vi "PM-A-Serial-test_setup.vi"() -> ()   [LabVIEW 2018]
uses:
  <vilib>/measure/matone.llb/Extract Single Tone Information 1 Chan.vi
  <vilib>/measure/NI_MAPro.lvlib
panel:
  out "Pulse":dbl format="%.2p"
  out "x-y":u32
  in  "sample rate [Hz] (1000)":dbl=1000.0
  out "error out":errorcluster
  out "Filter":waveform(dbl)(graph)
  in  "Addition signal to remove (0) [s]":dbl
  in  "Clear data":bool
  in  "Samples s":i32=10
  out "Raw":waveform(dbl)(graph)
  in  "Stop":bool
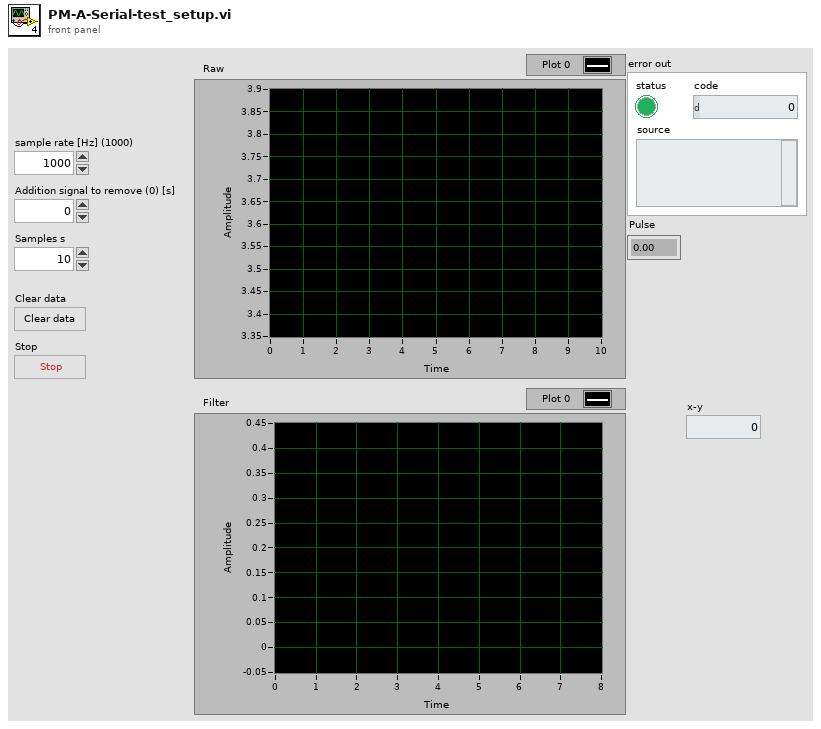
[diagram p1: front panel]
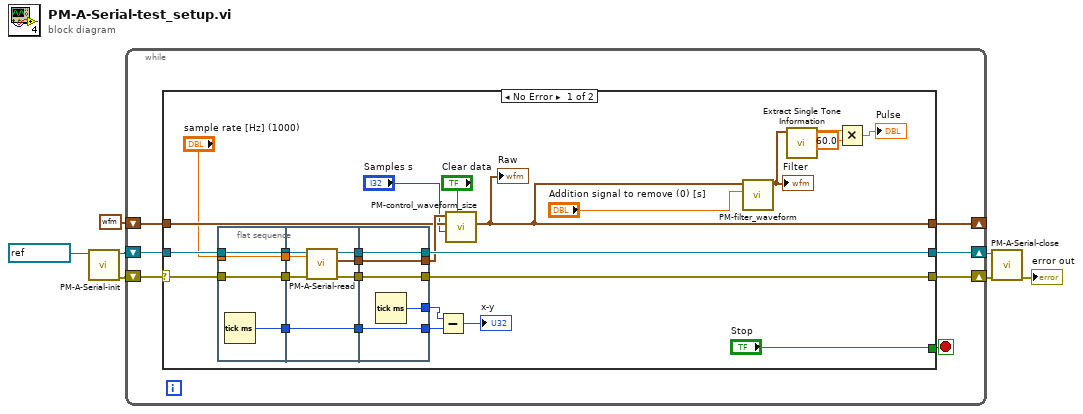
[diagram p0: block diagram]
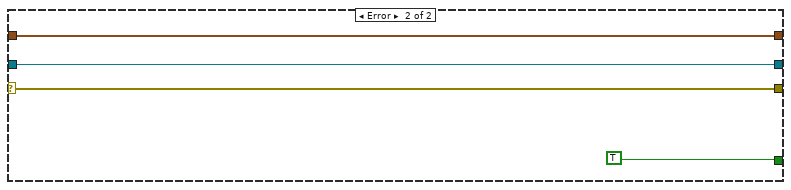
[diagram p2: hidden frame]
diagram:
  n1 = call "PM-A-Serial-init.vi"("VISA resource name"=refnum<visa-resource-name> "COM5" ("VISA resource name in")) -> ("error out"=w7:errorcluster, "VISA resource name out"=w6:refnum<visa-resource-name>)  [unwired: 9 in]
  n2 = while {
    shift-right: [w14] -> w2
    shift-left: w7 -> [w13]
    shift-right: [w12] -> w3
    shift-left: w6 -> [w11]
    shift-right: [w9] -> _
    shift-left: waveform(dbl) {"t0"=timestamp(0 s since 1904-01-01), "dt"=1.0, "Y"=[]} ("data") -> [w10]
    stop <- w8 stop-if-true
    n3 = case shown="No Error" w13 {
      selector: w13 -> [w32 w60]
      tunnel: [w33 w60] -> w14
      tunnel: [w31 w59] -> w12
      tunnel: w11 -> [w30 w59]
      tunnel: w10 -> [w28 w58]
      tunnel: [w19 w58] -> w9
      tunnel: ["Stop" TRUE ("Stop")] -> w8
      frame No Error {
        n4 = flat-sequence {
          tunnel: "sample rate [Hz] (1000)" -> [w43]
          tunnel: w30 -> [w44]
          tunnel: w32 -> [w45]
          tunnel: [w45] -> w41
          tunnel: [w44] -> w40
          tunnel: [w43] -> w39
          tunnel: [w42] -> w38
          tunnel: [w52] -> w37
          tunnel: [w50] -> w36
          tunnel: [w48] -> w35
          tunnel: w41 -> [w51]
          tunnel: w40 -> [w49]
          tunnel: w39 -> [w47]
          tunnel: [w46] -> w34
          tunnel: w38 -> [w46]
          tunnel: [w55] -> w29
          tunnel: [w56] -> w31
          tunnel: [w57] -> w33
          tunnel: w37 -> [w57]
          tunnel: w36 -> [w56]
          tunnel: w35 -> [w55]
          tunnel: [w54] -> w21
          tunnel: w34 -> [w54]
          tunnel: [w53] -> w22
          frame #0 {
            n5 = Tick Count (ms)() -> (millisecond timer value=w42:u32)
          }
          frame #1 {
            n6 = call "PM-A-Serial-read.vi"("sample rate [Hz] (1000)"=w47, "error in (no error)"=w51, "VISA resource name in"=w49) -> ("error out"=w52:errorcluster, "data"=w48:waveform(dbl), "VISA resource name out"=w50:refnum<visa-resource-name>)  [unwired: 6 in]
          }
          frame #2 {
            n7 = Tick Count (ms)() -> (millisecond timer value=w53:u32)
          }
        }
        n8 = Subtract(x=w22, y=w21) -> (x-y=→"x-y":u32)
        n9 = call "PM-control_waveform_size.vi"("Clear waveform"="Clear data", "Samples s"="Samples s", "old waveform"=w28, "New waveform"=w29) -> ("waveform"=w19:waveform(dbl))  [unwired: 7 in]
        "Raw" <- w19
        n10 = call "PM-filter_waveform.vi"("Addition signal to remove (0) [s]"="Addition signal to remove (0) [s]", "waveform in"=w19) -> ("waveform out"=w18:waveform(dbl))  [unwired: 8 in, 1 out]
        "Filter" <- w18
        n11 = call-poly <vilib>:"Extract Single Tone Information.vi"("time signal in"=w18) -> ("detected frequency"=w17:dbl)  [unwired: 5 in, 5 out]
        n12 = Multiply(x=w17, y=60.0) -> (x*y=→"Pulse":dbl)
      }
      frame Error {
      }
    }
  }
  n13 = call "PM-A-Serial-close.vi"("error in (no error)"=w2, "VISA resource name"=w3) -> ("error out"=→"error out":errorcluster)  [unwired: 9 in]
